vi "ParCreate.vi"(7 "Boolean":bool, 11 "error in (no error)":errorcluster) -> (4 "ref out":u64, 15 "error out":errorcluster)   [LabVIEW 2020, in "Snap7.lvlib"]
uses:
  Snap7.lvlib
  windows/lv_snap7.dll
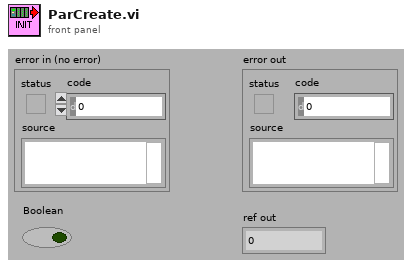
[diagram p1: front panel]
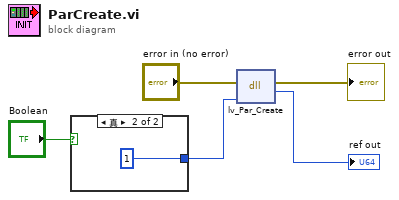
[diagram p0: block diagram]
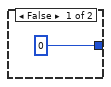
[diagram p2: hidden frame]
diagram:
  n1 = case shown="真" "Boolean" {
    tunnel: [0 1] -> w2
    frame False {
    }
    frame True {
    }
  }
  n2 = dll-call lib="PTH2fabs CUsersFeng项目HLCEPS300-2性能试验台SourcesSnap7libwindowslv_snap7.dll" fn="lv_Par_Create"(error in="error in (no error)", "Active"=w2) -> (error out=→"error out":errorcluster, "return type"=→"ref out":u64)  [unwired: 3 in, 1 out]
